vi "Initialize Status.vi"(8 "error in (no error)":errorcluster, 10 "Transfer Group Status":refnum<class "Status Pointer.lvclass">, 11 "Transfer Group in":refnum<class "Transfer Group.lvclass">) -> (0 "error out":errorcluster, 3 "Transfer Group out":refnum<class "Transfer Group.lvclass">)   [LabVIEW 2017, in "DSF Core.lvlib" / "Transfer Group.lvclass"]
uses:
  Transfer Group.lvclass
  Status/Status Pointer.lvclass
  C:/Program Files (x86)/National Instruments/LabVIEW 2017/vi.lib/NI/Memory Manager/Classes/Pointer/Pointer.lvclass
  <vilib>/NI/Memory Manager/Classes/Pointer/Pointer.lvclass/Pointer.ctl
  Transfer Group.lvclass/Transfer Group.ctl
  <vilib>/NI/Memory Manager/Classes/Pointer/Get Address.vi
  <vilib>/NI/Memory Manager/Classes/Pointer/Pointer.lvclass
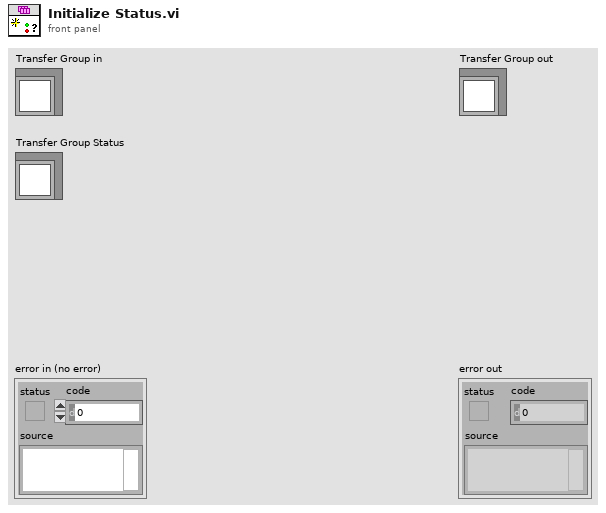
[diagram p1: front panel]
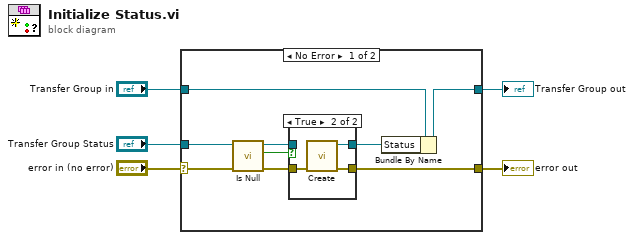
[diagram p0: block diagram]
diagram:
  n1 = case shown="No Error" "error in (no error)" {
    selector: "error in (no error)" -> [w7 w21]
    tunnel: [w6 w21] -> w4
    tunnel: [w13 w20] -> w2
    tunnel: "Transfer Group in" -> [w14 w20]
    tunnel: "Transfer Group Status" -> [w8 _]
    frame No Error {
      n2 = call <vilib>:"Is Null.vi"("error in (no error)"=w7, "Pointer in"=w8) -> ("error out"=w11:errorcluster, "null?"=w10:bool, "Pointer out"=w12:refnum<class "Status Pointer.lvclass">)  [unwired: 7 in]
      n3 = case shown="True" w10 {
        tunnel: w12 -> [w15 _]
        tunnel: [w15 w18] -> w9
        tunnel: w11 -> [w16 w19]
        tunnel: [w16 w17] -> w6
        frame False {
        }
        frame True {
          n4 = call "Create.vi"("error in (no error)"=w19) -> ("error out"=w17:errorcluster, "status pointer"=w18:refnum<class "Status Pointer.lvclass">)  [unwired: 9 in]
        }
      }
      n5 = Bundle By Name(cluster=w14, "Status"=w9) -> (w13:refnum<class "Transfer Group.lvclass">)
    }
    frame Error {
    }
  }
  "error out" <- w4
  "Transfer Group out" <- w2
